vi "image_processing.vi"(5 "NG_rules":T3, 7 "parameter":T2={"image imshow"=FALSE, "side length (mm)"=0.0, "Main Range (Threshold)"={"Lower value"=73.0, "Upper value"=255.0}, "side velocity threshold"=0.0, "Sub Range (Threshold)"={"Lower value"=73.0, "Upper value"=255.0}, "close kernel size"=0.0, "open kernel size"=0.0, "side angle offest (threshold)"=0.0}, 11 "image":T1(plugin-control)) -> (0 "PASS":bool, 2 "NG code":dbl, 3 "display image":T1(plugin-control))   [LabVIEW 2017]
uses:
  <vilib>/vision/NI_Vision_Development_Module.lvlib
panel:
  out "angle offset":dbl
  out "side angle offest":dbl
  out "side length (mm)":dbl
  out "ratio (cutting offest)":dbl
  out "damaged (mil)":dbl
  out "glitch (mil)":dbl
  out "open kernel size":dbl
  out "close kernel size":dbl
  in  "side velocity threshold":dbl
  out "Main Range (Threshold)":cluster{"Lower value":sgl, "Upper value":sgl}={"Lower value"=73.0, "Upper value"=255.0}
  out "image imshow":bool
  out "time image processing":u32
  out "time load image":u32
  out "Y Resolution":i32
  out "X Resolution":i32
  out "black image":T1(plugin-control)
  out "buffer image":T1(plugin-control)
  out "Sub Range (Threshold)":cluster{"Lower value":sgl, "Upper value":sgl}={"Lower value"=73.0, "Upper value"=255.0}
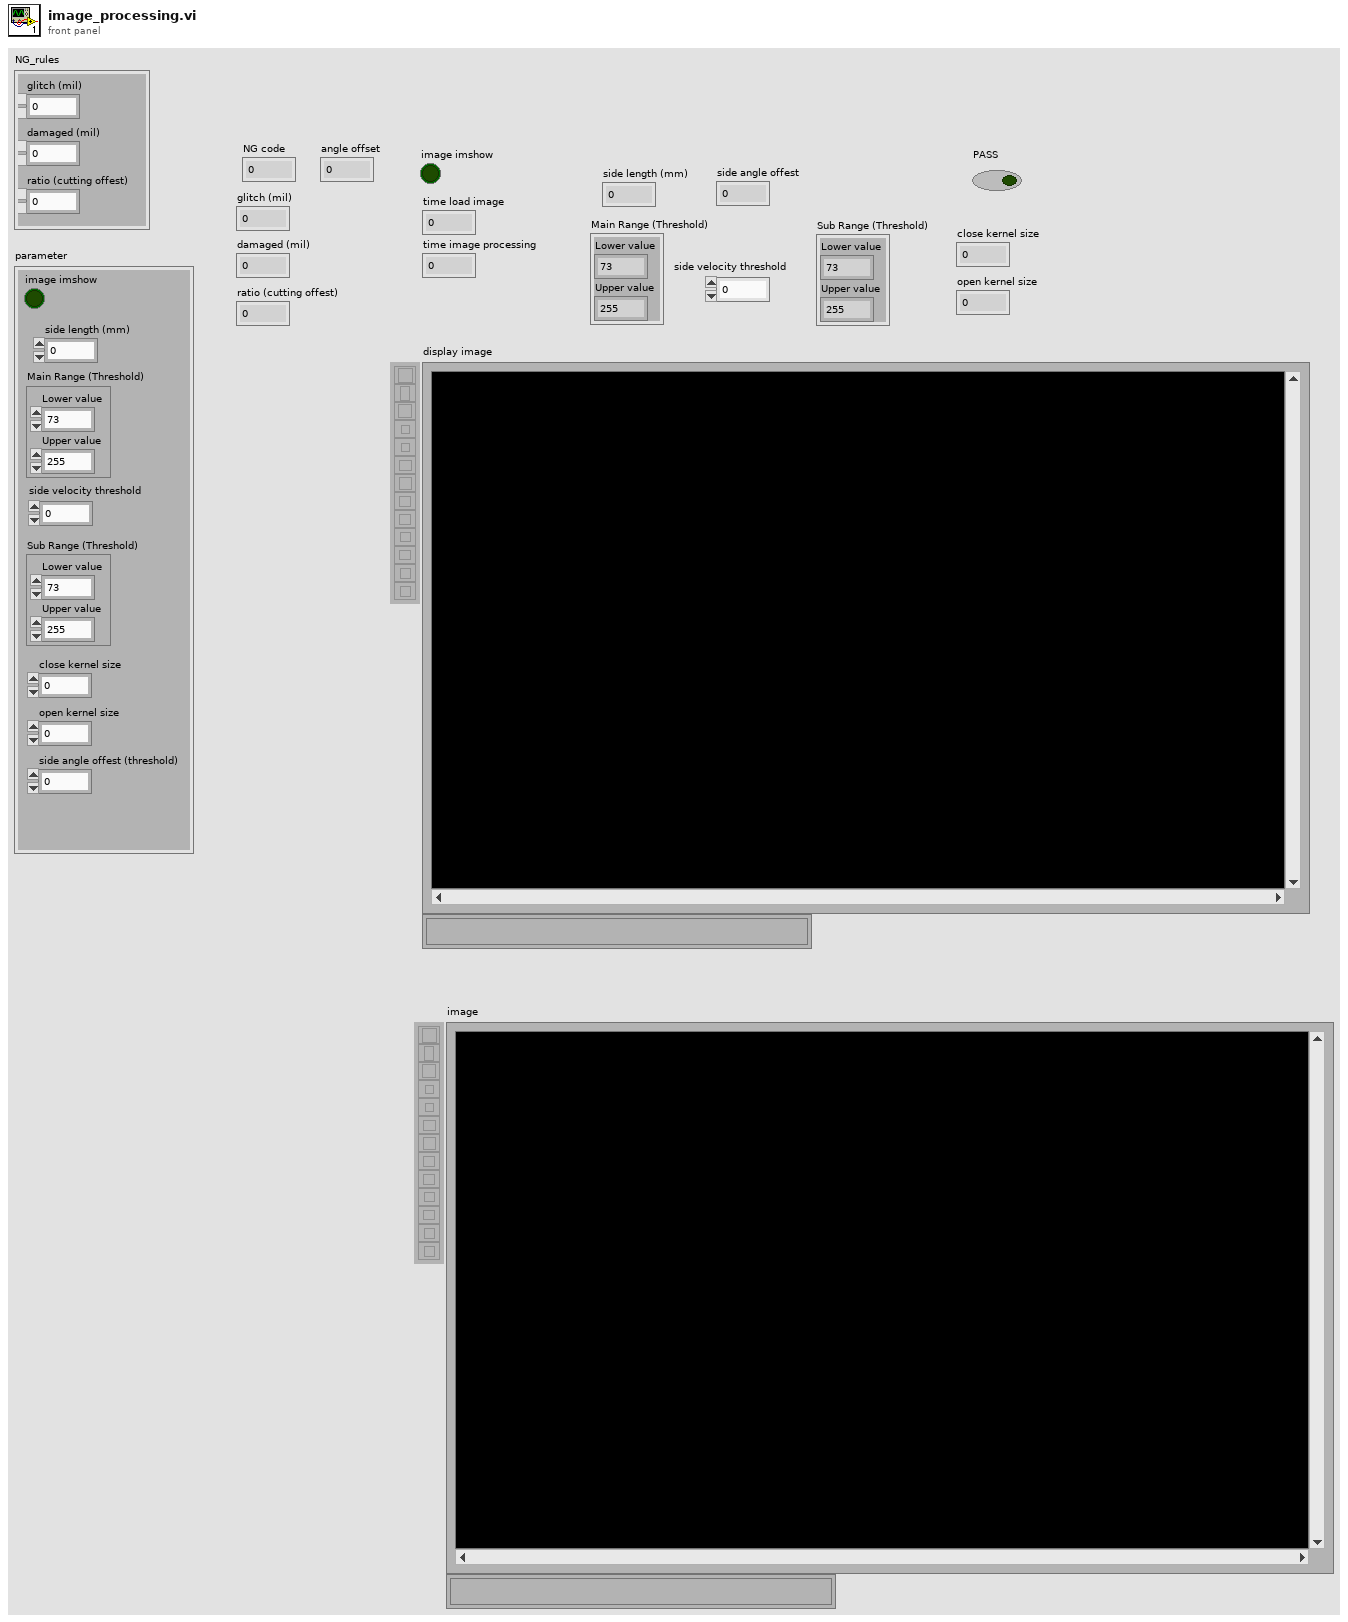
[diagram p1: front panel]
types:
  T1 = typedef "IMAQ Image.ctl" = refnum<image>
  T2 = cluster{"image imshow":bool, "side length (mm)":dbl, "Main Range (Threshold)":cluster{"Lower value":sgl, "Upper value":sgl}, "side velocity threshold":dbl, "Sub Range (Threshold)":cluster{"Lower value":sgl, "Upper value":sgl}, "close kernel size":dbl, "open kernel size":dbl, "side angle offest (threshold)":dbl}
  T3 = cluster{"glitch (mil)":dbl, "damaged (mil)":dbl, "ratio (cutting offest)":dbl}
  T4 = cluster{"Desired Font (Application)":enum16{"User-specified Font", "Application Font", "System Font", "Dialog Font"}, "[User-specified Font]":cluster{"Font Name":string, "Size":i16, "Strikeout?":bool, "Italic?":bool, "Underline?":bool, "Outline?":bool, "Shadow?":bool, "Bold?":bool, "Rotation Angle":dbl}, "Horizontal Alignment":i16, "Vertical Alignment":i16}
  T5 = enum32{"AutoM", "Close", "Dilate", "Erode", "Gradient", "Gradient out", "Gradient in", "Hit miss", "Open", "PClose", "POpen", "Thick", "Thin"}
  T6 = cluster{"Sigma":sgl, "HThresh":sgl, "LThres":sgl, "WindowSize":i32}
  T7 = cluster{"Number of Points":i32, "Open/Closed":i32, "Weight":dbl, "Contour Points":cluster{"X":dbl, "Y":dbl, "Curvature":dbl, "X Displacement":dbl, "Y Displacement":dbl}[]}[]
  T8 = cluster{"Left":i32, "Top":i32, "Right":i32, "Bottom":i32}
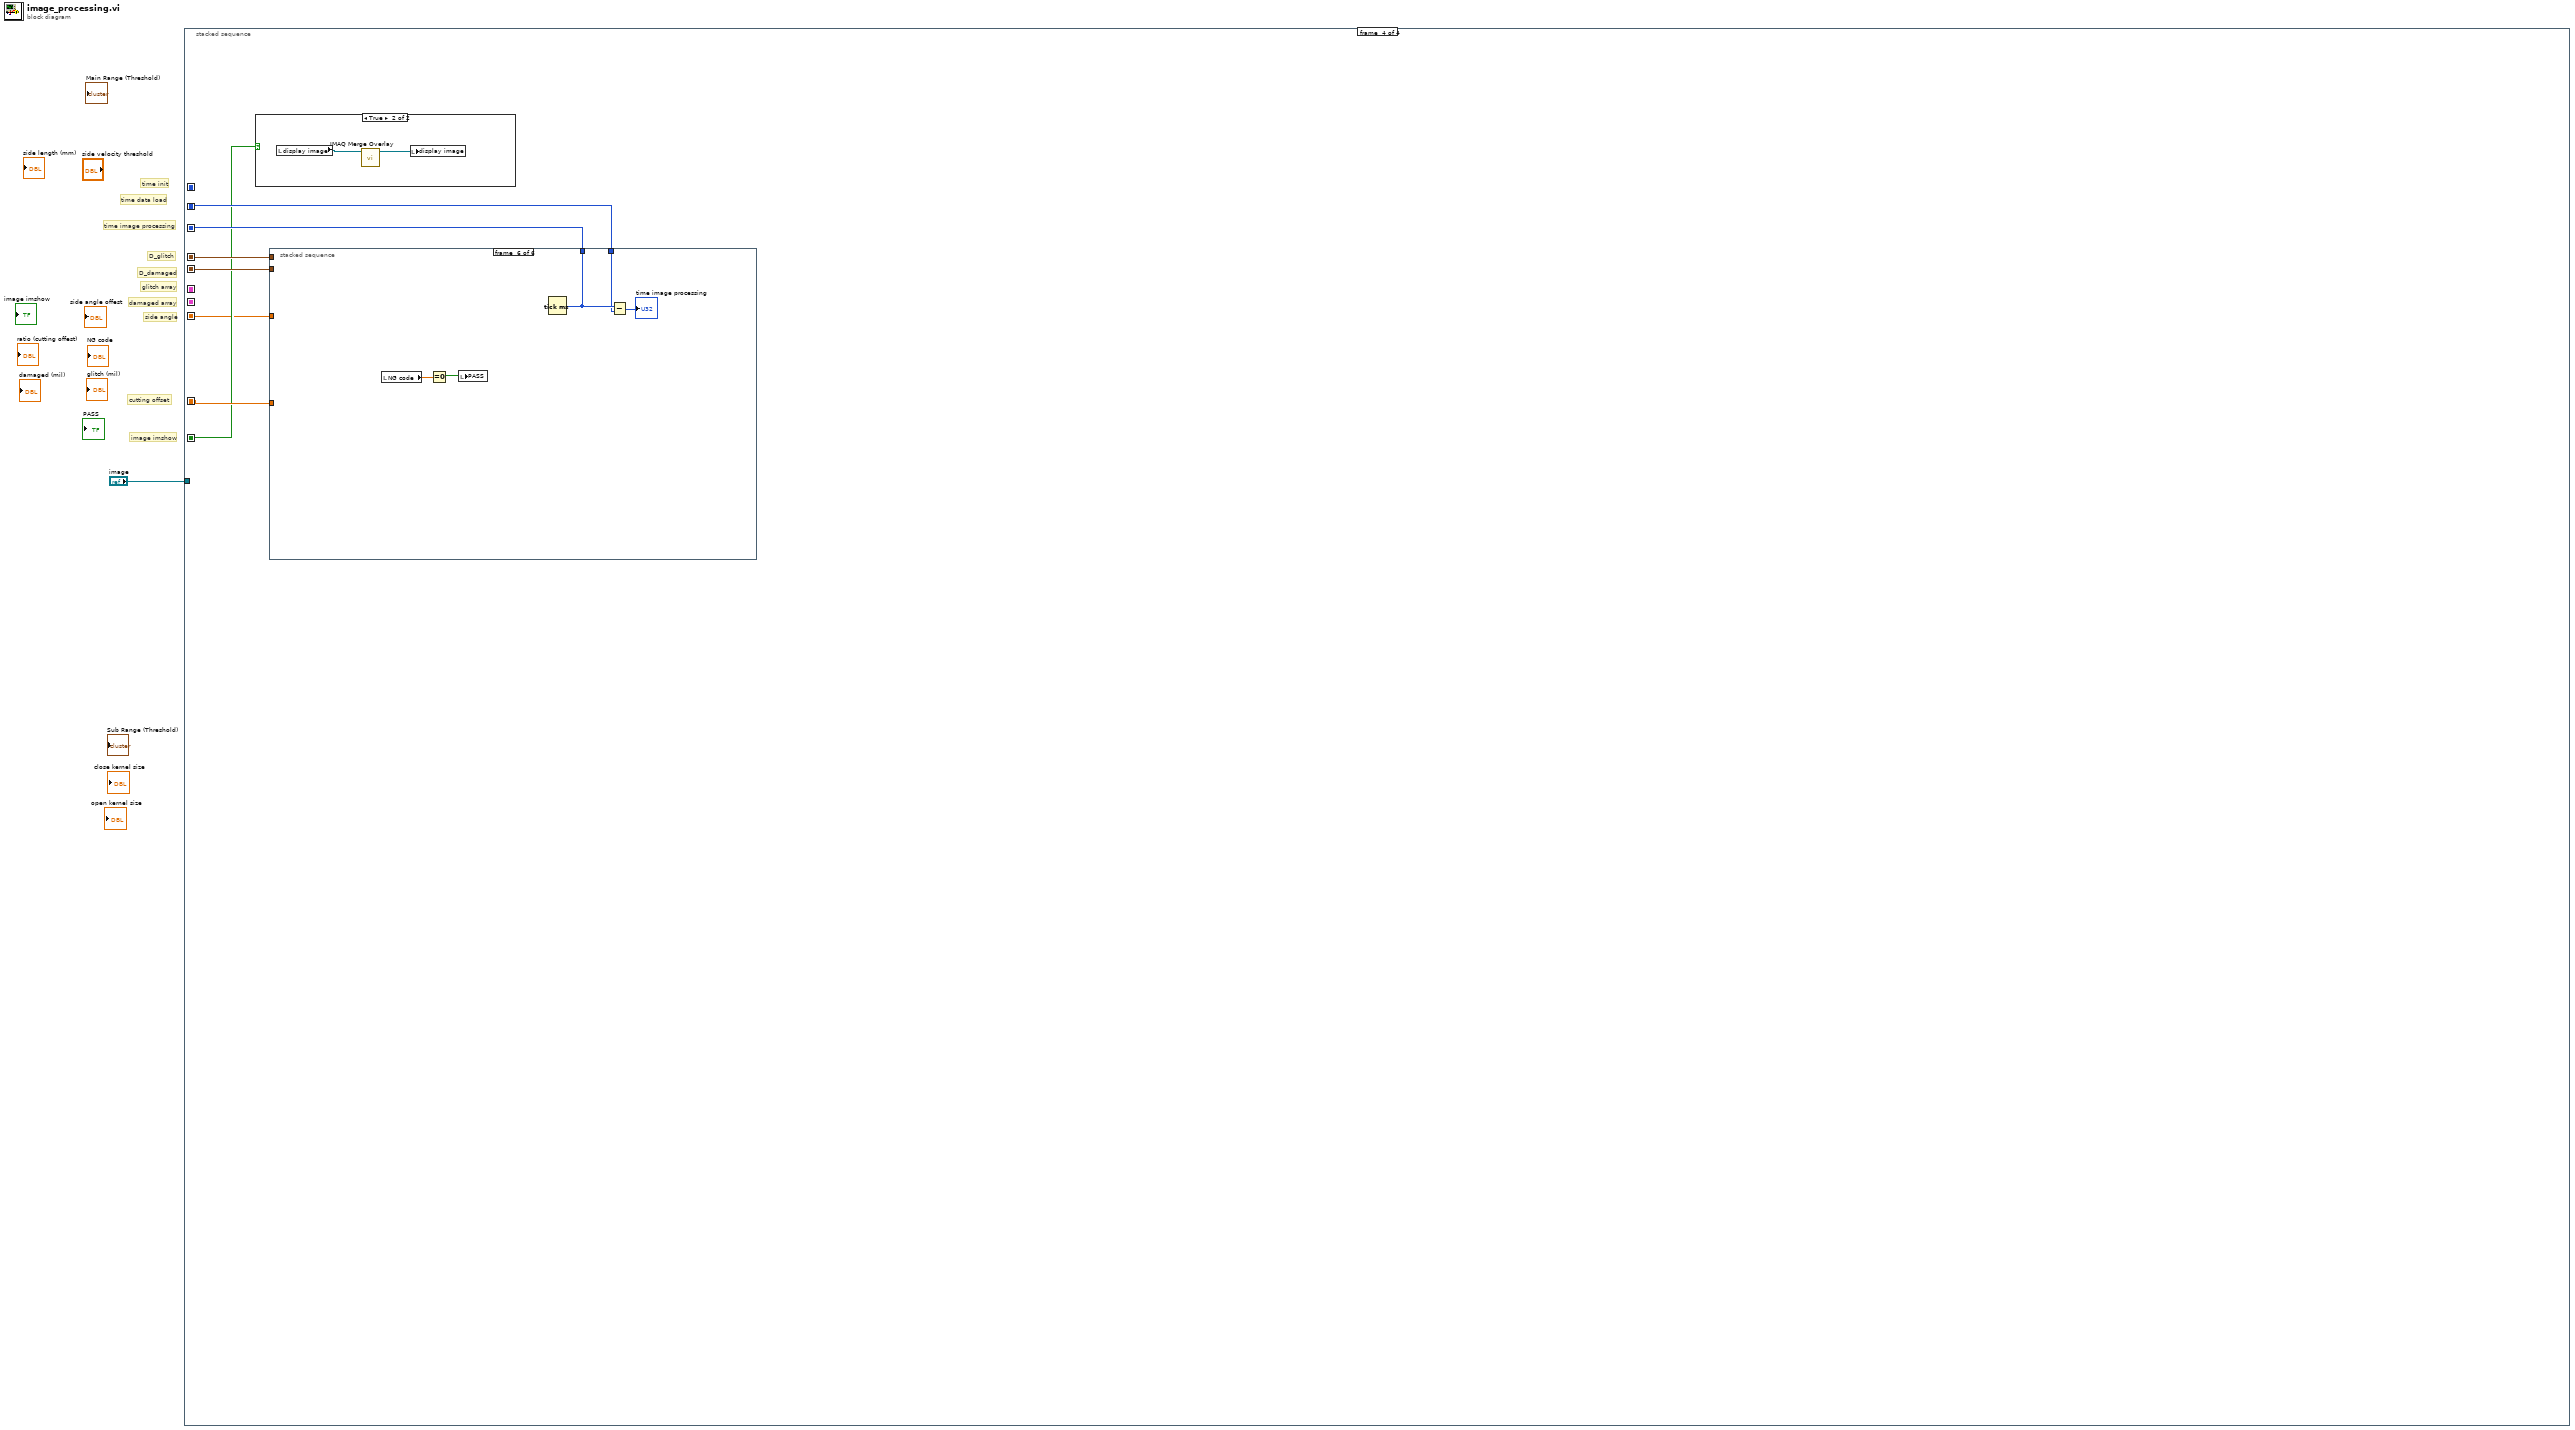
[diagram p0: block diagram]
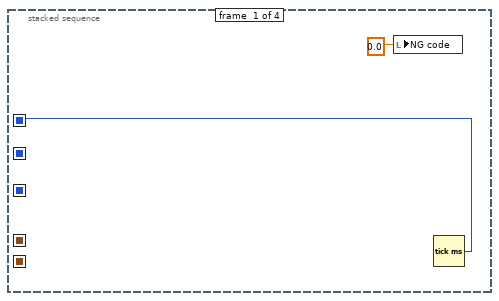
[diagram p2: hidden frame]
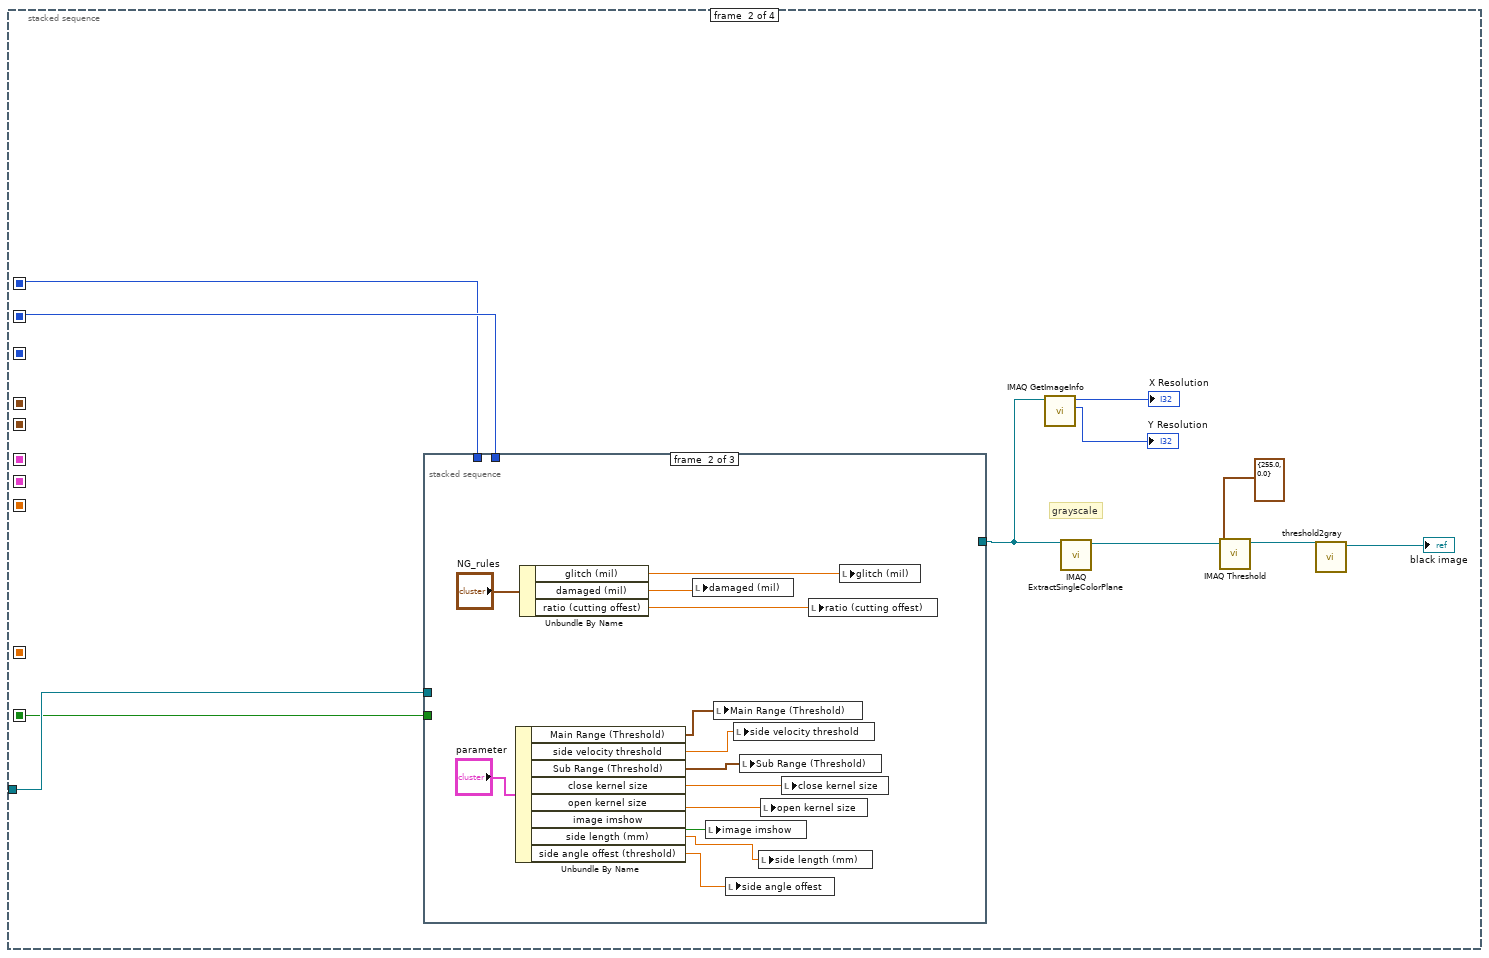
[diagram p3: hidden frame]
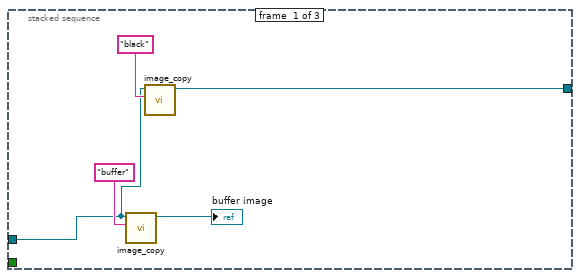
[diagram p4: hidden frame]
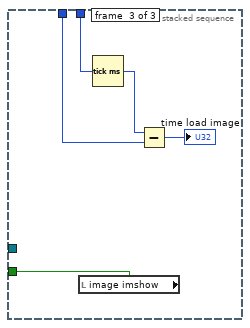
[diagram p5: hidden frame]
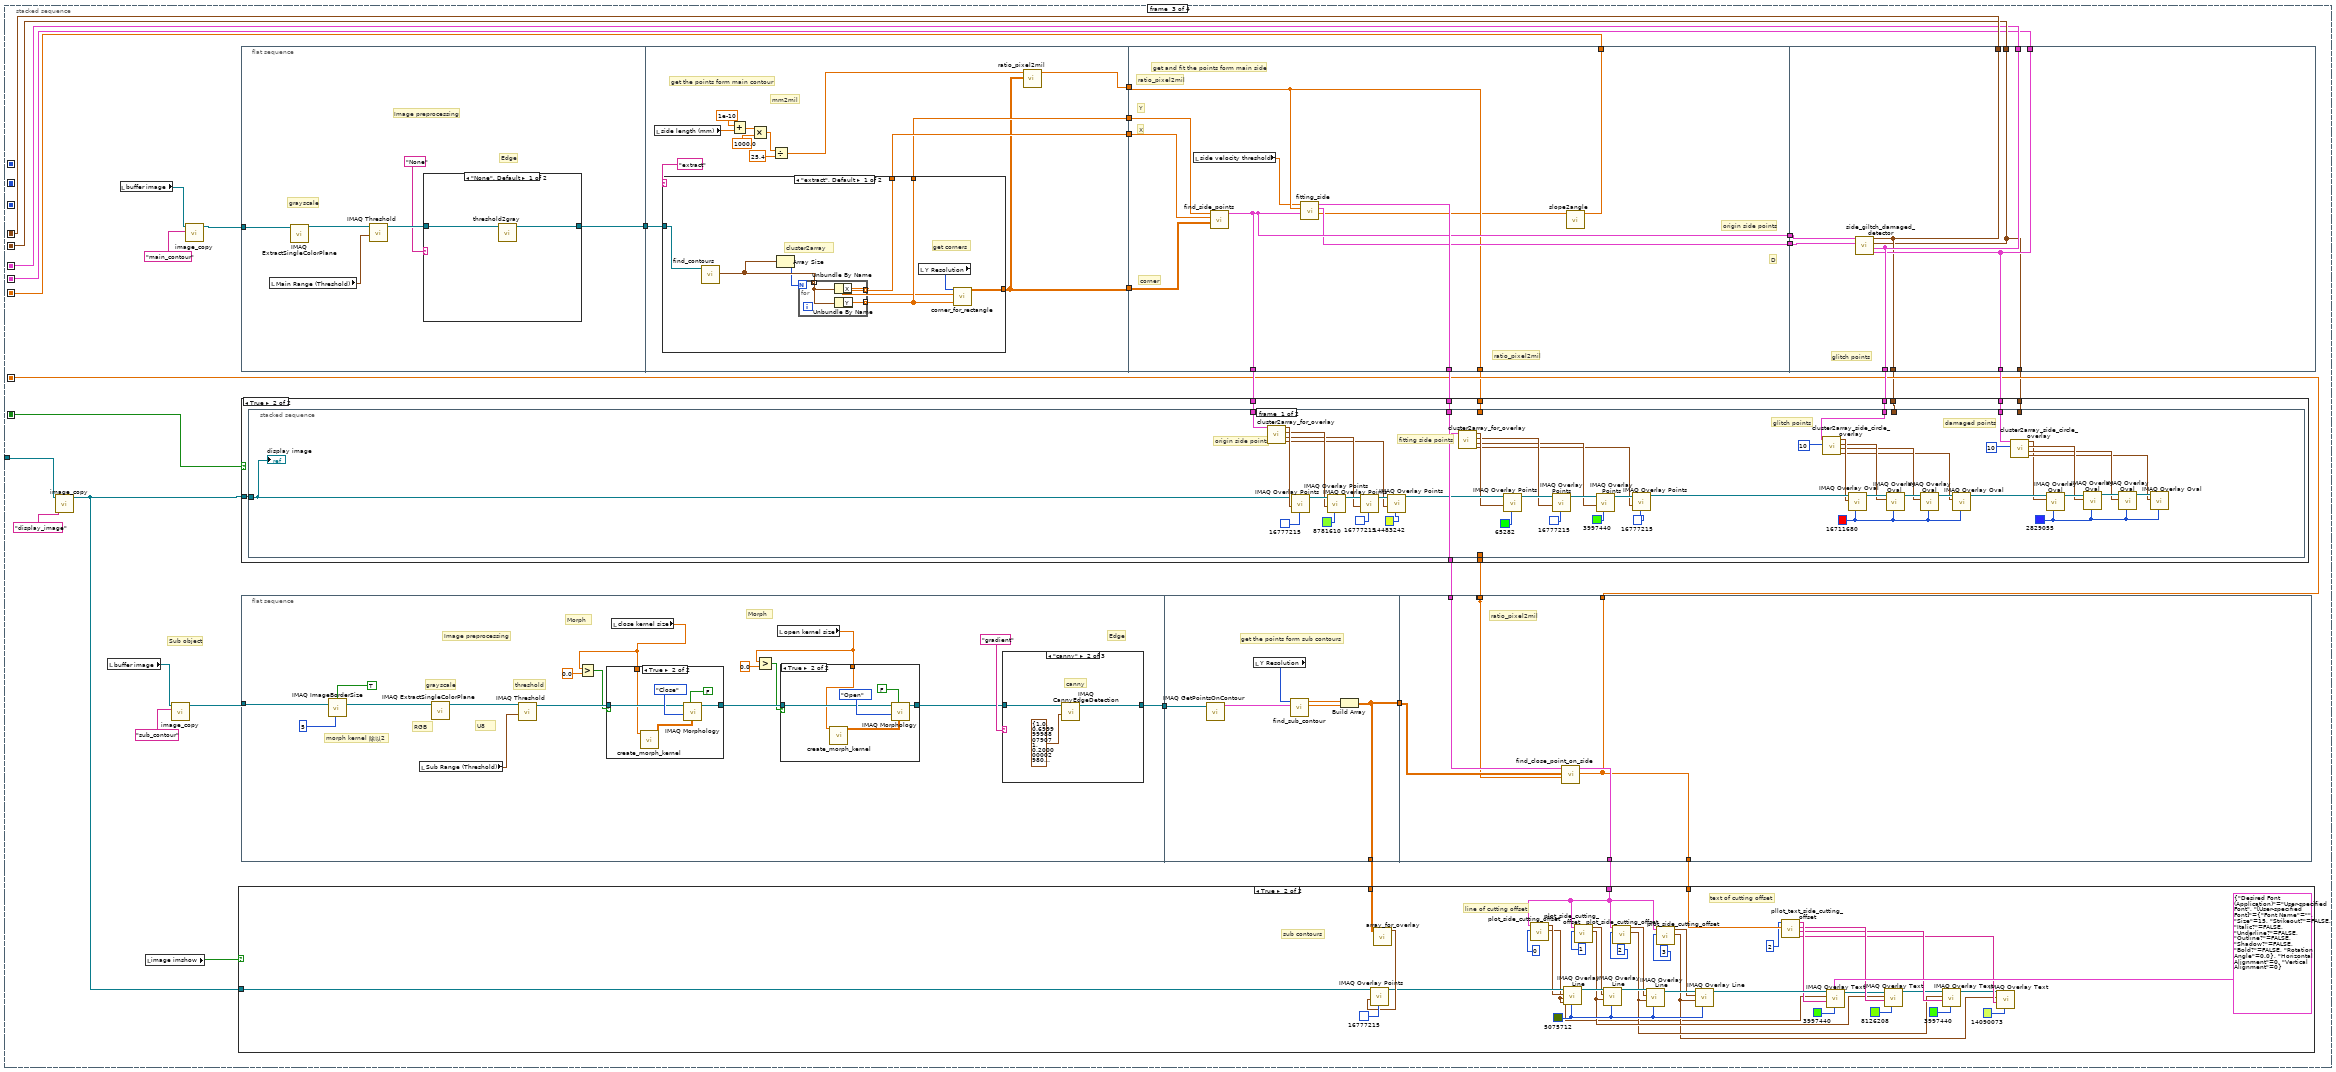
[diagram p6: hidden frame]
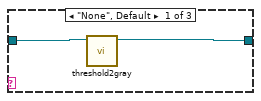
[diagram p10: hidden frame]
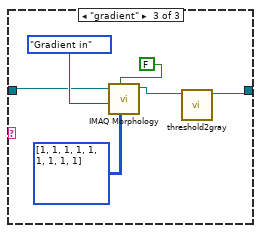
[diagram p11: hidden frame]
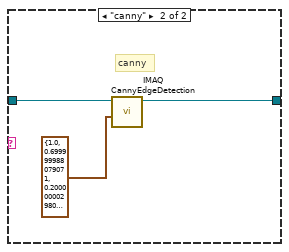
[diagram p12: hidden frame]
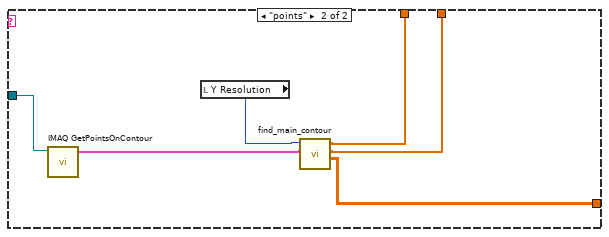
[diagram p13: hidden frame]
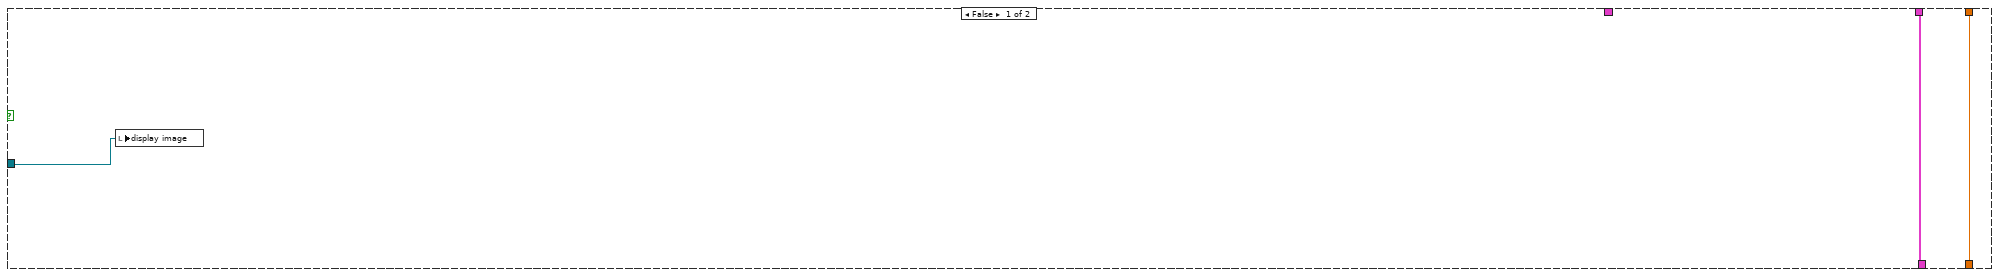
[diagram p14: hidden frame]
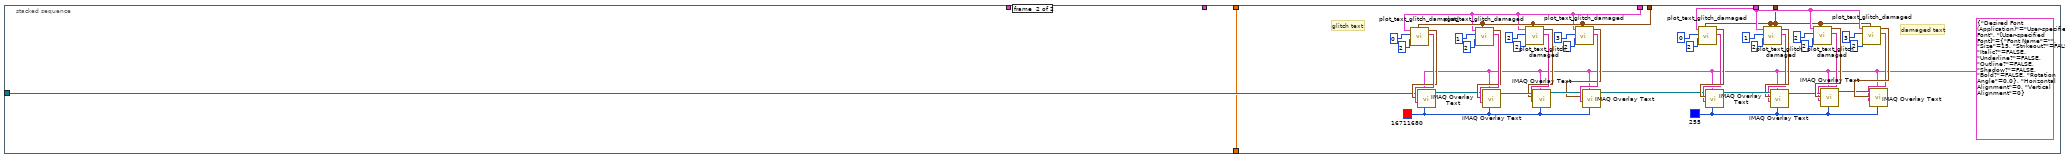
[diagram p15: hidden frame]
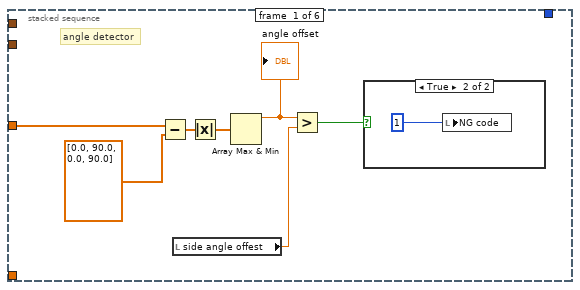
[diagram p17: hidden frame]
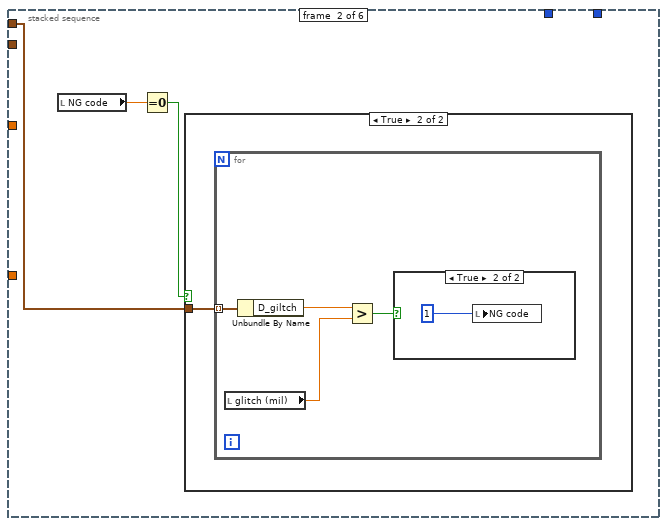
[diagram p19: hidden frame]
diagram:
  # "side angle"
  # "image imshow"
  # "cutting offset"
  # "damaged array"
  # "glitch array"
  # "D_damaged"
  # "D_glitch"
  # "time image processing"
  # "time data load"
  # "time init"
  n1 = stacked-sequence {
    seq-local: [w3 _ _ _] -> [_ w7 _ _]
    seq-local: [_ w8 _ _] -> [_ _ _ w334]
    seq-local: [_ _ _ w335] -> [_ _ _ _]
    seq-local: [_ _ w49 _] -> [_ _ _ w333]
    seq-local: [_ _ w48 _] -> [_ _ _ w332]
    seq-local: [_ _ w47 _] -> [_ _ _ _]
    seq-local: [_ _ w46 _] -> [_ _ _ _]
    seq-local: [_ _ w44 _] -> [_ _ _ w331]
    seq-local: [_ w4 _ _] -> [_ _ w38 w330]
    seq-local: [_ _ w37 _] -> [_ _ _ w329]
    tunnel: "image" -> [_ w9 w56 _]
    frame #0 {
      n2 = local write "NG code"(0.0 ("NG code")) -> ()
      n3 = Tick Count (ms)() -> (millisecond timer value=w3:u32)
    }
    frame #1 {
      # "grayscale"
      n4 = stacked-sequence {
        tunnel: [w17 _ _] -> w12
        tunnel: w9 -> [w16 _ _]
        tunnel: [_ _ w36] -> w8
        tunnel: w7 -> [_ _ w35]
        tunnel: [_ _ w33] -> w4
        frame #0 {
          n5 = call "image_copy.vi"("buffer name"="buffer" ("Image Name"), "image in"=w16) -> ("imgae out"=→"buffer image":T1)  [unwired: 9 in]
          n6 = call "image_copy.vi"("buffer name"="black" ("Image Name"), "image in"=w16) -> ("imgae out"=w17:T1)  [unwired: 9 in]
        }
        frame #1 {
          n7 = Unbundle By Name("parameter") -> ("Main Range (Threshold)"=w27:cluster{"Lower value":sgl, "Upper value":sgl}, "side velocity threshold"=w26:dbl, "Sub Range (Threshold)"=w25:cluster{"Lower value":sgl, "Upper value":sgl}, "close kernel size"=w24:dbl, "open kernel size"=w23:dbl, "image imshow"=w22:bool, "side length (mm)"=w21:dbl, "side angle offest (threshold)"=w20:dbl)
          n8 = Unbundle By Name("NG_rules") -> ("glitch (mil)"=w31:dbl, "damaged (mil)"=w30:dbl, "ratio (cutting offest)"=w29:dbl)
          n9 = local write "damaged (mil)"(w30) -> ()
          n10 = local write "image imshow"(w22) -> ()
          n11 = local write "Main Range (Threshold)"(w27) -> ()
          n12 = local write "side angle offest"(w20) -> ()
          n13 = local write "side velocity threshold"(w26) -> ()
          n14 = local write "Sub Range (Threshold)"(w25) -> ()
          n15 = local write "side length (mm)"(w21) -> ()
          n16 = local write "open kernel size"(w23) -> ()
          n17 = local write "close kernel size"(w24) -> ()
          n18 = local write "ratio (cutting offest)"(w29) -> ()
          n19 = local write "glitch (mil)"(w31) -> ()
        }
        frame #2 {
          n20 = local read "image imshow"() -> (w33:bool)
          n21 = Tick Count (ms)() -> (millisecond timer value=w36:u32)
          n22 = Subtract(x=w36, y=w35) -> (x-y=→"time load image":u32)
        }
      }
      n23 = call "IMAQ GetImageInfo"("Image"=w12) -> ("Y Resolution"=→"Y Resolution":i32, "X Resolution"=→"X Resolution":i32)  [unwired: 3 in, 6 out]
      n24 = call "IMAQ ExtractSingleColorPlane"("Image Src"=w12) -> ("Image Dst Out"=w14:T1)  [unwired: 3 in, 7 out]
      n25 = call "IMAQ Threshold"("Range"=cluster{"Lower value":sgl, "Upper value":sgl} {"Lower value"=255.0, "Upper value"=0.0}, "Image Src"=w14) -> ("Image Dst Out"=w6:T1)  [unwired: 4 in, 5 out]
      n26 = call "threshold2gray.vi"("threshold image"=w6) -> ("grayscale image"=→"black image":T1)  [unwired: 10 in]
    }
    frame #2 {
      # "Sub object"
      n27 = call "image_copy.vi"("buffer name"="display_image" ("Image Name"), "image in"=w56) -> ("imgae out"=w55:T1)  [unwired: 9 in]
      n28 = local read "buffer image"() -> (w65:T1)
      n29 = local read "buffer image"() -> (w73:T1)
      n30 = local read "image imshow"() -> (w52:bool)
      n31 = call "image_copy.vi"("buffer name"="sub_contour" ("Image Name"), "image in"=w65) -> ("imgae out"=w64:T1)  [unwired: 9 in]
      n32 = call "image_copy.vi"("buffer name"="main_contour" ("Image Name"), "image in"=w73) -> ("imgae out"=w72:T1)  [unwired: 9 in]
      n33 = case shown="True" w52 {
        tunnel: w55 -> [_ w109]
        tunnel: w54 -> [_ w108]
        tunnel: w53 -> [_ w99]
        tunnel: w43 -> [_ w91]
        frame False {
        }
        frame True {
          w103 = u32 5075712 ("Color")
          # "text of cutting offset"
          # "line of cutting offset"
          # "sub contours"
          n34 = call "array_for_overlay.vi"("Array in"=w108) -> ("Array out"=w110:cluster{"X":i32, "Y":i32}[])  [unwired: 10 in]
          n35 = call "IMAQ Overlay Points"("Color"=u32 16777215, "Array of Points"=w110, "Image"=w109) -> ("Image Out"=w107:T1)  [unwired: 7 in, 1 out]
          n36 = call "plot_side_cutting_offset.vi"("index"=0, "coord cluster"=w99) -> ("End Point out"=w75:cluster{"X":i32, "Y":i32}, "Start Point out"=w88:cluster{"X":i32, "Y":i32})  [unwired: 8 in]
          n37 = call "IMAQ Overlay Line"("Color"=w103, "End Point"=w75, "Start Point"=w88, "Image"=w107) -> ("Image Out"=w106:T1)  [unwired: 6 in, 1 out]
          n38 = call "plot_side_cutting_offset.vi"("index"=1, "coord cluster"=w99) -> ("End Point out"=w78:cluster{"X":i32, "Y":i32}, "Start Point out"=w93:cluster{"X":i32, "Y":i32})  [unwired: 8 in]
          n39 = call "IMAQ Overlay Line"("Color"=w103, "End Point"=w78, "Start Point"=w93, "Image"=w106) -> ("Image Out"=w105:T1)  [unwired: 6 in, 1 out]
          n40 = call "plot_side_cutting_offset.vi"("index"=2, "coord cluster"=w99) -> ("End Point out"=w77:cluster{"X":i32, "Y":i32}, "Start Point out"=w94:cluster{"X":i32, "Y":i32})  [unwired: 8 in]
          n41 = call "IMAQ Overlay Line"("Color"=w103, "End Point"=w77, "Start Point"=w94, "Image"=w105) -> ("Image Out"=w104:T1)  [unwired: 6 in, 1 out]
          n42 = call "plot_side_cutting_offset.vi"("index"=3, "coord cluster"=w99) -> ("End Point out"=w76:cluster{"X":i32, "Y":i32}, "Start Point out"=w95:cluster{"X":i32, "Y":i32})  [unwired: 8 in]
          n43 = call "IMAQ Overlay Line"("Color"=w103, "End Point"=w76, "Start Point"=w95, "Image"=w104) -> ("Image Out"=w97:T1)  [unwired: 6 in, 1 out]
          n44 = call "pllot_text_side_cutting_offset.vi"("D cutting offset array"=w91, "precision"=2 ("index")) -> ("Left side length"=w82:string, "Bottom side length"=w83:string, "Right side length"=w84:string, "Top side length"=w89:string)  [unwired: 6 in]
          n45 = call "IMAQ Overlay Text"("Text Color (black)"=u32 3997440, "Font, Size & Style"=T4 {"Desired Font (Application)"=enum."User-specified Font", "[User-specified Font]"={"Font Name"="", "Size"=15, "Strikeout?"=FALSE, "Italic?"=FALSE, "Underline?"=FALSE, "Outline?"=FALSE, "Shadow?"=FALSE, "Bold?"=FALSE, "Rotation Angle"=0.0}, "Horizontal Alignment"=0, "Vertical Alignment"=0}, "String"=w89, "Origin"=w75, "Image"=w97) -> ("Image Out"=w81:T1)  [unwired: 5 in, 1 out]
          n46 = call "IMAQ Overlay Text"("Text Color (black)"=u32 8126208, "String"=w84, "Origin"=w78, "Image"=w81) -> ("Image Out"=w80:T1)  [unwired: 6 in, 1 out]
          n47 = call "IMAQ Overlay Text"("Text Color (black)"=u32 3997440, "String"=w83, "Origin"=w77, "Image"=w80) -> ("Image Out"=w79:T1)  [unwired: 6 in, 1 out]
          n48 = call "IMAQ Overlay Text"("Text Color (black)"=u32 14090073, "String"=w82, "Origin"=w76, "Image"=w79) -> ()  [unwired: 6 in, 2 out]
        }
      }
      n49 = flat-sequence {
        tunnel: w72 -> [w170]
        tunnel: [w167] -> w71
        tunnel: w71 -> [w187]
        tunnel: [w181] -> w70
        tunnel: [w186] -> w68
        tunnel: [w185] -> w67
        tunnel: [w179] -> w59
        tunnel: w70 -> [w214]
        tunnel: [w210] -> w69
        tunnel: w68 -> [w213]
        tunnel: w67 -> [w212]
        tunnel: [w211] -> w62
        tunnel: w59 -> [w208]
        tunnel: [w210] -> w51
        tunnel: [w209] -> w50
        tunnel: [w208] -> w40
        tunnel: [w205] -> w37
        tunnel: [w218] -> w61
        tunnel: [w217] -> w60
        tunnel: w51 -> [w220]
        tunnel: w50 -> [w219]
        tunnel: [w218] -> w47
        tunnel: [w217] -> w46
        tunnel: [w216] -> w49
        tunnel: [w215] -> w48
        tunnel: [w216] -> w42
        tunnel: [w215] -> w41
        frame #0 {
          # "Image preprocessing"
          # "grayscale"
          # "Edge"
          n50 = local read "Main Range (Threshold)"() -> (w165:cluster{"Lower value":sgl, "Upper value":sgl})
          n51 = call "IMAQ ExtractSingleColorPlane"("Image Src"=w170) -> ("Image Dst Out"=w169:T1)  [unwired: 3 in, 7 out]
          n52 = call "IMAQ Threshold"("Range"=w165, "Image Src"=w169) -> ("Image Dst Out"=w168:T1)  [unwired: 4 in, 5 out]
          n53 = case shown="\"None\", Default" "None" {
            tunnel: [w171 w175] -> w167
            tunnel: w168 -> [w172 w174]
            frame "None", Default {
              n54 = call "threshold2gray.vi"("threshold image"=w172) -> ("grayscale image"=w171:T1)  [unwired: 10 in]
            }
            frame "canny" {
              # "canny"
              n55 = call "IMAQ CannyEdgeDetection"("Image Src"=w174, "Filter Parameters"=T6 {"Sigma"=1.0, "HThresh"=0.7, "LThres"=0.2, "WindowSize"=9}) -> ("Image Dst Out"=w175:T1)  [unwired: 2 in, 5 out]
            }
          }
        }
        frame #1 {
          # "mm2mil"
          # "get the points form main contour"
          n56 = local read "side length (mm)"() -> (w176:dbl)
          n57 = case shown="\"extract\", Default" "extract" {
            tunnel: w187 -> [w191 w204]
            tunnel: [w192 w199] -> w181
            tunnel: [w190 w200] -> w185
            tunnel: [w189 w201] -> w186
            frame "extract", Default {
              # "get corners"
              # "cluster2array"
              n58 = call "find_contours.vi"("image in"=w191) -> ("Source Image Points"=w195:cluster{"X":dbl, "Y":dbl}[])  [unwired: 9 in, 1 out]
              n59 = Array Size(array=w195) -> (size(s)=w193:i32)
              n60 = for {
                N: w193 -> [_]
                tunnel: w195 -> [w197] mode=indexing
                tunnel: [w198] -> w189 mode=indexing
                tunnel: [w196] -> w190 mode=indexing
                n61 = Unbundle By Name(w197) -> ("X"=w198:dbl)
                n62 = Unbundle By Name(w197) -> ("Y"=w196:dbl)
              }
              n63 = local read "Y Resolution"() -> (w194:i32)
              n64 = call "corner_for_rectangle.vi"("Y"=w190, "X"=w189, "Y Resolution"=w194) -> ("corner"=w192:dbl[][])  [unwired: 7 in, 1 out]
            }
            frame "points" {
              n65 = call "IMAQ GetPointsOnContour"("Image (Edge Image)"=w204) -> ("Segment Information"=w202:T7)  [unwired: 3 in, 2 out]
              n66 = local read "Y Resolution"() -> (w203:i32)
              n67 = call "find_main_contour.vi"("Segment Information"=w202, "Y Resolution"=w203) -> ("max corner"=w199:dbl[][], "Y"=w200:dbl[], "X"=w201:dbl[])  [unwired: 7 in]
            }
          }
          n68 = Add(x=1e-10, y=w176) -> (x+y=w177:dbl)
          n69 = Multiply(x=w177, y=1000.0) -> (x*y=w183:dbl)
          n70 = Divide(x=w183, y=25.4) -> (x/y=w180:dbl)
          n71 = call "ratio_pixel2mil.vi"("max corner in"=w181, "side length (mm)"=w180) -> ("ratio"=w179:dbl)  [unwired: 9 in]
        }
        frame #2 {
          # "ratio_pixel2mil"
          # "origin side points"
          # "D"
          # "corner"
          # "X"
          # "Y"
          # "ratio_pixel2mil"
          # "get and fit the points form main side"
          n72 = local read "side velocity threshold"() -> (w207:dbl)
          n73 = call "find_side_points.vi"("corner"=w214, "X  coords array"=w213, "Y coords array"=w212) -> ("side of clusters"=w210:cluster{"Array out":dbl[][]}[])  [unwired: 8 in]
          n74 = call "fitting_side.vi"("side of clusters"=w210, "ratio"=w208, "side velocity threshold"=w207) -> ("slope array"=w206:dbl[], "D of clusters"=w209:cluster{"D":ext[]}[], "fitting clusters"=w211:cluster{"fitting array":dbl[][]}[])  [unwired: 6 in]
          n75 = call "slope2angle.vi"("slope array"=w206) -> ("x/y"=w205:dbl[])  [unwired: 10 in]
        }
        frame #3 {
          # "glitch points"
          n76 = call "side_giltch_damaged_detector.vi"("D of clusters"=w219, "side of clusters"=w220) -> ("damaged clusters"=w217:cluster{"damaged coord":dbl[]}[], "giltch of clusters"=w218:cluster{"giltch_coord":dbl[]}[], "D damaged of clusters"=w215:cluster{"D_damaged":ext}[], "D giltch of clusters"=w216:cluster{"D_giltch":ext}[])  [unwired: 6 in]
        }
      }
      n77 = flat-sequence {
        tunnel: w64 -> [w125]
        tunnel: [w121] -> w63
        tunnel: w63 -> [w159]
        tunnel: [w154] -> w58
        tunnel: [w154] -> w54
        tunnel: w58 -> [w164]
        tunnel: [w163] -> w53
        tunnel: w45 -> [w162]
        tunnel: [w160] -> w44
        tunnel: [w160] -> w43
        tunnel: [w161] -> _
        tunnel: w39 -> [w161]
        frame #0 {
          # "Morph"
          # "Image preprocessing"
          # "Morph"
          # "morph kernel 除以2"
          # "Edge"
          # "U8"
          # "RGB"
          # "threshold"
          # "grayscale"
          n78 = call "IMAQ ImageBorderSize"("Get/Set Status? (Set)"=TRUE, "Image"=w125, "Image border size in"=5) -> ("Image Out"=w124:T1)  [unwired: 1 in, 2 out]
          n79 = local read "Sub Range (Threshold)"() -> (w114:cluster{"Lower value":sgl, "Upper value":sgl})
          n80 = call "IMAQ ExtractSingleColorPlane"("Image Src"=w124) -> ("Image Dst Out"=w128:T1)  [unwired: 3 in, 7 out]
          n81 = call "IMAQ Threshold"("Range"=w114, "Image Src"=w128) -> ("Image Dst Out"=w126:T1)  [unwired: 4 in, 5 out]
          n82 = local read "close kernel size"() -> (w113:dbl)
          n83 = Greater?(x=w113, y=0.0) -> (0:w118:bool)
          n84 = case shown="True" w118 {
            tunnel: w126 -> [w136 w141]
            tunnel: [w136 w140] -> w119
            tunnel: w113 -> [_ w139]
            frame False {
            }
            frame True {
              n85 = call "create_morph_kernel.vi"("kernel size"=w139) -> ("kernel"=w138:dbl[][])  [unwired: 10 in]
              n86 = call "IMAQ Morphology"("Structuring Element"=w138, "Square/Hexa (Square)"=FALSE, "Operation"=T5."Close", "Image Src"=w141) -> ("Image Dst Out"=w140:T1)  [unwired: 3 in, 4 out]
            }
          }
          n87 = local read "open kernel size"() -> (w112:dbl)
          n88 = Greater?(x=w112, y=0.0) -> (0:w115:bool)
          n89 = case shown="True" w115 {
            tunnel: [w129 w134] -> w120
            tunnel: w119 -> [w129 w133]
            tunnel: w112 -> [_ w130]
            frame False {
            }
            frame True {
              n90 = call "create_morph_kernel.vi"("kernel size"=w130) -> ("kernel"=w131:dbl[][])  [unwired: 10 in]
              n91 = call "IMAQ Morphology"("Structuring Element"=w131, "Square/Hexa (Square)"=FALSE, "Operation"=T5."Open", "Image Src"=w133) -> ("Image Dst Out"=w134:T1)  [unwired: 3 in, 4 out]
            }
          }
          n92 = case shown="\"canny\"" "gradient" {
            tunnel: [w143 w147 w148] -> w121
            tunnel: w120 -> [w144 w146 w150]
            frame "None", Default {
              n93 = call "threshold2gray.vi"("threshold image"=w144) -> ("grayscale image"=w143:T1)  [unwired: 10 in]
            }
            frame "canny" {
              # "canny"
              n94 = call "IMAQ CannyEdgeDetection"("Image Src"=w146, "Filter Parameters"=T6 {"Sigma"=1.0, "HThresh"=0.7, "LThres"=0.2, "WindowSize"=9}) -> ("Image Dst Out"=w147:T1)  [unwired: 2 in, 5 out]
            }
            frame "gradient" {
              n95 = call "IMAQ Morphology"("Structuring Element"=i32[][] [[1, 1, 1], [1, 1, 1], [1, 1, 1]], "Square/Hexa (Square)"=FALSE, "Operation"=T5."Gradient in", "Image Src"=w150) -> ("Image Dst Out"=w149:T1)  [unwired: 3 in, 4 out]
              n96 = call "threshold2gray.vi"("threshold image"=w149) -> ("grayscale image"=w148:T1)  [unwired: 10 in]
            }
          }
        }
        frame #1 {
          # "get the points form sub contours"
          n97 = call "IMAQ GetPointsOnContour"("Image (Edge Image)"=w159) -> ("Segment Information"=w158:T7)  [unwired: 3 in, 2 out]
          n98 = local read "Y Resolution"() -> (w157:i32)
          n99 = call "find_sub_contour.vi"("Segment Information"=w158, "Y Resolution"=w157) -> ("Y"=w155:dbl[], "X"=w156:dbl[])  [unwired: 8 in]
          n100 = Build Array(w156, w155) -> (w154:dbl[][])
        }
        frame #2 {
          # "ratio_pixel2mil"
          n101 = call "find_close_point_on_side.vi"("ratio_pixel2mil"=w161, "Array"=w164, "fitting clusters"=w162) -> ("D cutting offset array"=w160:ext[], "coord cluster"=w163:cluster{dbl[][]}[])  [unwired: 7 in]
        }
      }
      n102 = case shown="True" w38 {
        tunnel: w55 -> [w221 w232]
        tunnel: w69 -> [_ w231]
        tunnel: w62 -> [w223 w228]
        tunnel: w61 -> [_ w229]
        tunnel: w60 -> [_ w230]
        tunnel: [w223 w228] -> w45
        tunnel: w42 -> [_ w227]
        tunnel: w41 -> [_ w226]
        tunnel: w40 -> [w222 w225]
        tunnel: [w222 w224] -> w39
        frame False {
          n103 = local write "display image"(w221) -> ()
        }
        frame True {
          n104 = stacked-sequence {
            tunnel: w232 -> [w233 w324]
            tunnel: w231 -> [w255 _]
            tunnel: w230 -> [w240 w287]
            tunnel: w229 -> [w235 w309]
            tunnel: w228 -> [w234 _]
            tunnel: w227 -> [_ w311]
            tunnel: w226 -> [_ w286]
            tunnel: w225 -> [_ w281]
            tunnel: [_ w281] -> w224
            frame #0 {
              w257 = u32 2829055 ("Color")
              w258 = u32 16711680 ("Color")
              # "damaged points"
              # "glitch points"
              # "fitting side points"
              # "origin side points"
              n105 = call "cluster2array_for_overlay.vi"("side of clusters"=w255) -> ("Left side points"=w251:cluster{"X":i32, "Y":i32}[], "Bottom side points"=w252:cluster{"X":i32, "Y":i32}[], "Right side points"=w253:cluster{"X":i32, "Y":i32}[], "Top side points"=w254:cluster{"X":i32, "Y":i32}[])  [unwired: 7 in]
              n106 = call "IMAQ Overlay Points"("Color"=u32 16777215, "Array of Points"=w254, "Image"=w233) -> ("Image Out"=w277:T1)  [unwired: 7 in, 1 out]
              n107 = call "IMAQ Overlay Points"("Color"=u32 8781610, "Array of Points"=w253, "Image"=w277) -> ("Image Out"=w279:T1)  [unwired: 7 in, 1 out]
              n108 = call "IMAQ Overlay Points"("Color"=u32 16777215, "Array of Points"=w252, "Image"=w279) -> ("Image Out"=w278:T1)  [unwired: 7 in, 1 out]
              n109 = call "IMAQ Overlay Points"("Color"=u32 14483242, "Array of Points"=w251, "Image"=w278) -> ("Image Out"=w266:T1)  [unwired: 7 in, 1 out]
              n110 = call "cluster2array_for_overlay.vi"("side of clusters"=w234) -> ("Left side points"=w247:cluster{"X":i32, "Y":i32}[], "Bottom side points"=w248:cluster{"X":i32, "Y":i32}[], "Right side points"=w249:cluster{"X":i32, "Y":i32}[], "Top side points"=w250:cluster{"X":i32, "Y":i32}[])  [unwired: 7 in]
              n111 = call "IMAQ Overlay Points"("Color"=u32 65282, "Array of Points"=w250, "Image"=w266) -> ("Image Out"=w270:T1)  [unwired: 7 in, 1 out]
              n112 = call "IMAQ Overlay Points"("Color"=u32 16777215, "Array of Points"=w249, "Image"=w270) -> ("Image Out"=w268:T1)  [unwired: 7 in, 1 out]
              n113 = call "IMAQ Overlay Points"("Color"=u32 3997440, "Array of Points"=w248, "Image"=w268) -> ("Image Out"=w269:T1)  [unwired: 7 in, 1 out]
              n114 = call "IMAQ Overlay Points"("Color"=u32 16777215, "Array of Points"=w247, "Image"=w269) -> ("Image Out"=w256:T1)  [unwired: 7 in, 1 out]
              n115 = call "cluster2array_side_circle_overlay.vi"("radius"=10 ("index"), "giltch of clusters"=w235) -> ("Left side points"=w243:T8, "Bottom side points"=w244:T8, "Right side points"=w245:T8, "Top side points"=w246:T8)  [unwired: 6 in]
              n116 = call "IMAQ Overlay Oval"("Color"=w258, "Bounding Rectangle"=w246, "Image"=w256) -> ("Image Out"=w265:T1)  [unwired: 7 in, 1 out]
              n117 = call "IMAQ Overlay Oval"("Color"=w258, "Bounding Rectangle"=w245, "Image"=w265) -> ("Image Out"=w264:T1)  [unwired: 7 in, 1 out]
              n118 = call "IMAQ Overlay Oval"("Color"=w258, "Bounding Rectangle"=w244, "Image"=w264) -> ("Image Out"=w263:T1)  [unwired: 7 in, 1 out]
              n119 = call "IMAQ Overlay Oval"("Color"=w258, "Bounding Rectangle"=w243, "Image"=w263) -> ("Image Out"=w259:T1)  [unwired: 7 in, 1 out]
              n120 = call "cluster2array_side_circle_overlay.vi"("radius"=10 ("index"), "giltch of clusters"=w240) -> ("Left side points"=w237:T8, "Bottom side points"=w238:T8, "Right side points"=w239:T8, "Top side points"=w236:T8)  [unwired: 6 in]
              n121 = call "IMAQ Overlay Oval"("Color"=w257, "Bounding Rectangle"=w236, "Image"=w259) -> ("Image Out"=w260:T1)  [unwired: 7 in, 1 out]
              n122 = call "IMAQ Overlay Oval"("Color"=w257, "Bounding Rectangle"=w239, "Image"=w260) -> ("Image Out"=w261:T1)  [unwired: 7 in, 1 out]
              n123 = call "IMAQ Overlay Oval"("Color"=w257, "Bounding Rectangle"=w238, "Image"=w261) -> ("Image Out"=w262:T1)  [unwired: 7 in, 1 out]
              n124 = call "IMAQ Overlay Oval"("Color"=w257, "Bounding Rectangle"=w237, "Image"=w262) -> ()  [unwired: 7 in, 2 out]
              "display image" <- w233
            }
            frame #1 {
              w283 = u32 255 ("Text Color (black)")
              w285 = T4 {"Desired Font (Application)"=enum."User-specified Font", "[User-specified Font]"={"Font Name"="", "Size"=15, "Strikeout?"=FALSE, "Italic?"=FALSE, "Underline?"=FALSE, "Outline?"=FALSE, "Shadow?"=FALSE, "Bold?"=FALSE, "Rotation Angle"=0.0}, "Horizontal Alignment"=0, "Vertical Alignment"=0} ("Font, Size & Style")
              w284 = u32 16711680 ("Text Color (black)")
              # "damaged text"
              # "glitch text"
              n125 = call "plot_text_glitch_damaged.vi"("D of clusters"=w311, "precision"=2 ("index (page)"), "index"=0 ("index (page)"), "array clusters"=w309) -> ("string"=w326:string, "Origin"=w325:cluster{"X":i32, "Y":i32})  [unwired: 6 in]
              n126 = call "IMAQ Overlay Text"("Text Color (black)"=w284, "Font, Size & Style"=w285, "String"=w326, "Origin"=w325, "Image"=w324) -> ("Image Out"=w319:T1)  [unwired: 5 in, 1 out]
              n127 = call "plot_text_glitch_damaged.vi"("D of clusters"=w311, "precision"=2 ("index (page)"), "index"=1 ("index (page)"), "array clusters"=w309) -> ("string"=w323:string, "Origin"=w320:cluster{"X":i32, "Y":i32})  [unwired: 6 in]
              n128 = call "IMAQ Overlay Text"("Text Color (black)"=w284, "Font, Size & Style"=w285, "String"=w323, "Origin"=w320, "Image"=w319) -> ("Image Out"=w312:T1)  [unwired: 5 in, 1 out]
              n129 = call "plot_text_glitch_damaged.vi"("D of clusters"=w311, "precision"=2 ("index (page)"), "index"=2 ("index (page)"), "array clusters"=w309) -> ("string"=w316:string, "Origin"=w307:cluster{"X":i32, "Y":i32})  [unwired: 6 in]
              n130 = call "IMAQ Overlay Text"("Text Color (black)"=w284, "Font, Size & Style"=w285, "String"=w316, "Origin"=w307, "Image"=w312) -> ("Image Out"=w310:T1)  [unwired: 5 in, 1 out]
              n131 = call "plot_text_glitch_damaged.vi"("D of clusters"=w311, "precision"=2 ("index (page)"), "index"=3 ("index (page)"), "array clusters"=w309) -> ("string"=w315:string, "Origin"=w308:cluster{"X":i32, "Y":i32})  [unwired: 6 in]
              n132 = call "IMAQ Overlay Text"("Text Color (black)"=w284, "Font, Size & Style"=w285, "String"=w315, "Origin"=w308, "Image"=w310) -> ("Image Out"=w282:T1)  [unwired: 5 in, 1 out]
              n133 = call "plot_text_glitch_damaged.vi"("D of clusters"=w286, "precision"=2 ("index (page)"), "index"=0 ("index (page)"), "array clusters"=w287) -> ("string"=w290:string, "Origin"=w291:cluster{"X":i32, "Y":i32})  [unwired: 6 in]
              n134 = call "IMAQ Overlay Text"("Text Color (black)"=w283, "Font, Size & Style"=w285, "String"=w290, "Origin"=w291, "Image"=w282) -> ("Image Out"=w296:T1)  [unwired: 5 in, 1 out]
              n135 = call "plot_text_glitch_damaged.vi"("D of clusters"=w286, "precision"=2 ("index (page)"), "index"=1 ("index (page)"), "array clusters"=w287) -> ("string"=w292:string, "Origin"=w295:cluster{"X":i32, "Y":i32})  [unwired: 6 in]
              n136 = call "IMAQ Overlay Text"("Text Color (black)"=w283, "Font, Size & Style"=w285, "String"=w292, "Origin"=w295, "Image"=w296) -> ("Image Out"=w303:T1)  [unwired: 5 in, 1 out]
              n137 = call "plot_text_glitch_damaged.vi"("D of clusters"=w286, "precision"=2 ("index (page)"), "index"=2 ("index (page)"), "array clusters"=w287) -> ("string"=w299:string, "Origin"=w306:cluster{"X":i32, "Y":i32})  [unwired: 6 in]
              n138 = call "IMAQ Overlay Text"("Text Color (black)"=w283, "Font, Size & Style"=w285, "String"=w299, "Origin"=w306, "Image"=w303) -> ("Image Out"=w304:T1)  [unwired: 5 in, 1 out]
              n139 = call "plot_text_glitch_damaged.vi"("D of clusters"=w286, "precision"=2 ("index (page)"), "index"=3 ("index (page)"), "array clusters"=w287) -> ("string"=w300:string, "Origin"=w305:cluster{"X":i32, "Y":i32})  [unwired: 6 in]
              n140 = call "IMAQ Overlay Text"("Text Color (black)"=w283, "Font, Size & Style"=w285, "String"=w300, "Origin"=w305, "Image"=w304) -> ()  [unwired: 5 in, 2 out]
            }
          }
        }
      }
    }
    frame #3 {
      n141 = case shown="True" w330 {
        frame False {
        }
        frame True {
          n142 = local read "display image"() -> (w337:T1)
          n143 = call "IMAQ Merge Overlay"("Image Src"=w337) -> ("Image Dst Out"=w336:T1)  [unwired: 9 in, 1 out]
          n144 = local write "display image"(w336) -> ()
        }
      }
      n145 = stacked-sequence {
        tunnel: [_ _ _ _ _ w401] -> w335
        tunnel: w334 -> [_ _ _ _ _ w400]
        tunnel: w333 -> [_ w348 _ _ _ _]
        tunnel: w332 -> [_ _ w355 _ _ _]
        tunnel: w331 -> [_ _ _ w364 _ _]
        tunnel: w329 -> [w344 _ _ _ _ _]
        frame #0 {
          # "angle detector"
          n146 = Subtract(x=w344, y=dbl[] [0.0, 90.0, 0.0, 90.0] ("x/y")) -> (x-y=w342:dbl[])
          n147 = local read "side angle offest"() -> (w340:dbl)
          n148 = Absolute Value(x=w342) -> (abs(x)=w341:dbl[])
          n149 = Array Max & Min(array=w341) -> (max value=w339:dbl)  [unwired: 3 out]
          "angle offset" <- w339
          n150 = Greater?(x=w339, y=w340) -> (0:w338:bool)
          n151 = case shown="True" w338 {
            frame False {
            }
            frame True {
              n152 = local write "NG code"(1) -> ()
            }
          }
        }
        frame #1 {
          n153 = local read "NG code"() -> (w347:dbl)
          n154 = Equal To 0?(x=w347) -> (x = 0?=w346:bool)
          n155 = case shown="True" w346 {
            tunnel: w348 -> [_ w349]
            frame False {
            }
            frame True {
              n156 = for {
                tunnel: w349 -> [w353] mode=indexing
                n157 = local read "glitch (mil)"() -> (w350:dbl)
                n158 = Unbundle By Name(w353) -> ("D_giltch"=w352:ext)
                n159 = Greater?(x=w352, y=w350) -> (0:w351:bool)
                n160 = case shown="True" w351 {
                  frame False {
                  }
                  frame True {
                    n161 = local write "NG code"(1) -> ()
                  }
                }
              }
            }
          }
        }
        frame #2 {
          n162 = local read "NG code"() -> (w357:dbl)
          n163 = Equal To 0?(x=w357) -> (x = 0?=w356:bool)
          n164 = case shown="True" w356 {
            tunnel: w355 -> [_ w358]
            frame False {
            }
            frame True {
              n165 = for {
                tunnel: w358 -> [w361] mode=indexing
                n166 = local read "damaged (mil)"() -> (w359:dbl)
                n167 = Unbundle By Name(w361) -> ("D_damaged"=w362:ext)
                n168 = Greater?(x=w362, y=w359) -> (0:w360:bool)
                n169 = case shown="True" w360 {
                  frame False {
                  }
                  frame True {
                    n170 = local write "NG code"(3) -> ()
                  }
                }
              }
            }
          }
        }
        frame #3 {
          n171 = local read "NG code"() -> (w366:dbl)
          n172 = Equal To 0?(x=w366) -> (x = 0?=w365:bool)
          n173 = case shown="False" w365 {
            tunnel: w364 -> [_ w384]
            frame False {
            }
            frame True {
              n174 = Index Array(array=w384, index=2) -> (element=w380:ext)
              n175 = Index Array(array=w384, index=3) -> (element=w378:ext)
              n176 = Index Array(array=w384, index=0) -> (element=w381:ext)
              n177 = Index Array(array=w384, index=1) -> (element=w379:ext)
              n178 = Divide(x=w381, y=w380) -> (x/y=w375:ext)
              n179 = Divide(x=w379, y=w378) -> (x/y=w372:ext)
              n180 = Decrement(x=w372) -> (x-1=w373:ext)
              n181 = Decrement(x=w375) -> (x-1=w377:ext)
              n182 = Greater Than 0?(x=w373) -> (x > 0?=w374:bool)
              n183 = Greater Than 0?(x=w377) -> (x > 0?=w376:bool)
              n184 = local read "ratio (cutting offest)"() -> (w367:dbl)
              n185 = case shown="True" w374 {
                tunnel: w372 -> [w389 w391]
                tunnel: [w389 w390] -> w369
                frame False {
                }
                frame True {
                  n186 = Reciprocal(x=w391) -> (1/x=w390:ext)
                }
              }
              n187 = case shown="True" w376 {
                tunnel: w375 -> [w392 w394]
                tunnel: [w392 w393] -> w371
                frame False {
                }
                frame True {
                  n188 = Reciprocal(x=w394) -> (1/x=w393:ext)
                }
              }
              n189 = Less?(x=w371, y=w367) -> (x < y?=w370:bool)
              n190 = Less?(x=w369, y=w367) -> (x < y?=w368:bool)
              n191 = case shown="True" w370 {
                frame False {
                }
                frame True {
                  n192 = local write "NG code"(4) -> ()
                }
              }
              n193 = case shown="True" w368 {
                frame False {
                }
                frame True {
                  n194 = local write "NG code"(4) -> ()
                }
              }
            }
          }
        }
        frame #4 {
          n195 = local read "NG code"() -> (w396:dbl)
          n196 = Equal To 0?(x=w396) -> (x = 0?=w395:bool)
          n197 = case shown="True" w395 {
            frame False {
            }
            frame True {
            }
          }
        }
        frame #5 {
          n198 = local read "NG code"() -> (w398:dbl)
          n199 = Equal To 0?(x=w398) -> (x = 0?=w397:bool)
          n200 = local write "PASS"(w397) -> ()
          n201 = Tick Count (ms)() -> (millisecond timer value=w401:u32)
          n202 = Subtract(x=w401, y=w400) -> (x-y=→"time image processing":u32)
        }
      }
    }
  }
